vi "AddNumbers.vi"(10 "B":dbl, 11 "A":dbl) -> (2 "String":string, 3 "Sum":dbl)   [LabVIEW 2011]
panel:
  # "This VI is in the Math DLL Example\nbuild specification"
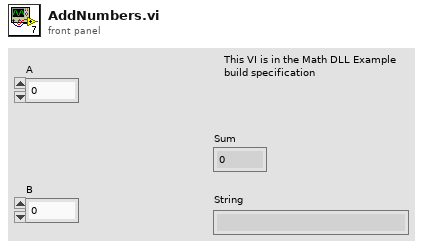
[diagram p1: front panel]
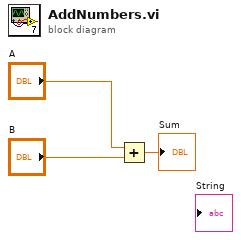
[diagram p0: block diagram]
diagram:
  n1 = Add(x="A", y="B") -> (x+y=→"Sum":dbl)
